vi "Configure Marker.vi"(6 "X-axis Position (0)":dbl, 7 "Peak Threshold (10%)":i32=10, 8 "error in (no error)":errorcluster, 9 "Marker Position (0: Maximum)":u16(ring) items=["Maximum", "Left of Maximum", "Right of Maximum", "X-axis Position"], 10 "Marker Number (1)":i32=1, 11 "VISA resource name":refnum<visa-resource-name>) -> (0 "error out":errorcluster, 3 "VISA resource name out":refnum<visa-resource-name>)   [LabVIEW 2015, in "Template - Spectrum Analyzer.lvlib"]
doc: "Configures the marker settings on the spectrum analyzer."
uses:
  <instrlib>/_Template - Spectrum Analyzer/Template - Spectrum Analyzer.lvlib
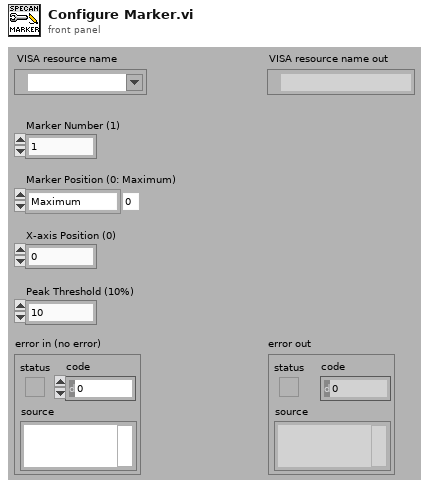
[diagram p1: front panel]
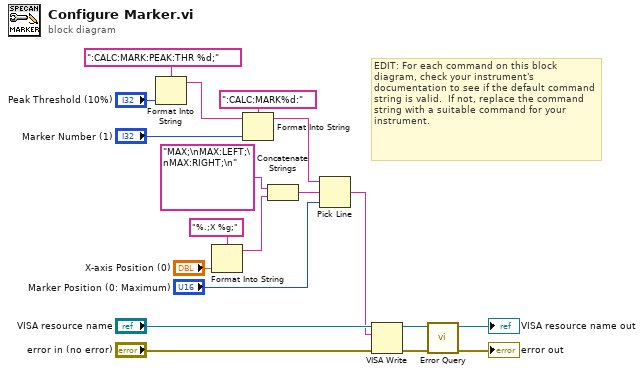
[diagram p0: block diagram]
diagram:
  # "EDIT: For each command on this block diagram, check your instrument's documentation to see if the default command  string is valid.  If not, replace the command string with a suitable command for your instrument."
  n1 = Format Into String(format string=":CALC:MARK:PEAK:THR %d;", "Peak Threshold (10%)") -> (resulting string=w11:string)  [unwired: 2 in, 1 out]
  n2 = Format Into String(format string="%.;X %g;", "X-axis Position (0)") -> (resulting string=w15:string)  [unwired: 2 in, 1 out]
  n3 = Format Into String(format string=":CALC:MARK%d:" ("initial string"), initial string=w11, "Marker Number (1)") -> (resulting string=w6:string)  [unwired: 1 in, 1 out]
  n4 = Concatenate Strings("MAX;\nMAX:LEFT;\nMAX:RIGHT;\n" ("multi-line string"), w15) -> (w13:string)
  n5 = Pick Line(string ("")=w6, multi-line string=w13, line index="Marker Position (0: Maximum)") -> (output string=w5:string)
  n6 = VISA Write(VISA resource name="VISA resource name", write buffer=w5, error in (no error)="error in (no error)") -> (VISA resource name out=w4:refnum<visa-resource-name>, error out=w2:errorcluster)  [unwired: 1 out]
  n7 = call <instrlib>:"Error Query.vi"("error in (no error)"=w2, "VISA resource name"=w4) -> ("error out"=→"error out":errorcluster, "VISA resource name out"=→"VISA resource name out":refnum<visa-resource-name>)  [unwired: 6 in, 2 out]
